vi "Get Square Periphery.vi"(9 "Radius":dbl=1.0, 10 "Neuron Position":i32[](array[numeric])=[3, 2, 7], 11 "Grid Size":i32[](array[numeric])=[10, 10, 10]) -> (3 "Square Periphery":i32[](array[numeric]))   [LabVIEW 2013]
doc: "This algorithm searches for the periphery of the input neuron given the position (x0,y0,z0) and the radius (r) of the neuron.\n The periphery is a square of edge length 6*r. It returns the ids of all the nodes inside the periphery. It takes into acount the limits of the grid (city).\n It includes the id of the node under study"
panel:
  out "No Elements Inside Periphery":i32
  out "Cycles":i32[](array[numeric])
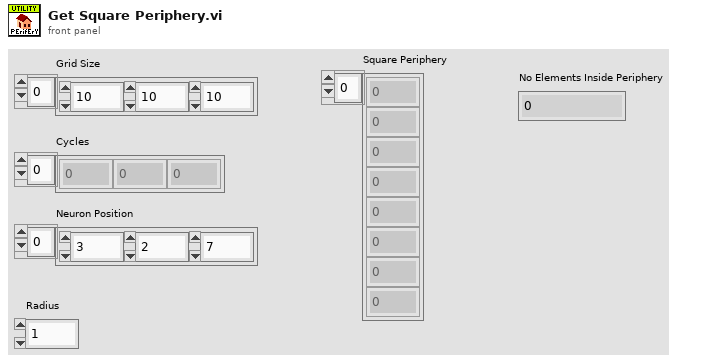
[diagram p1: front panel]
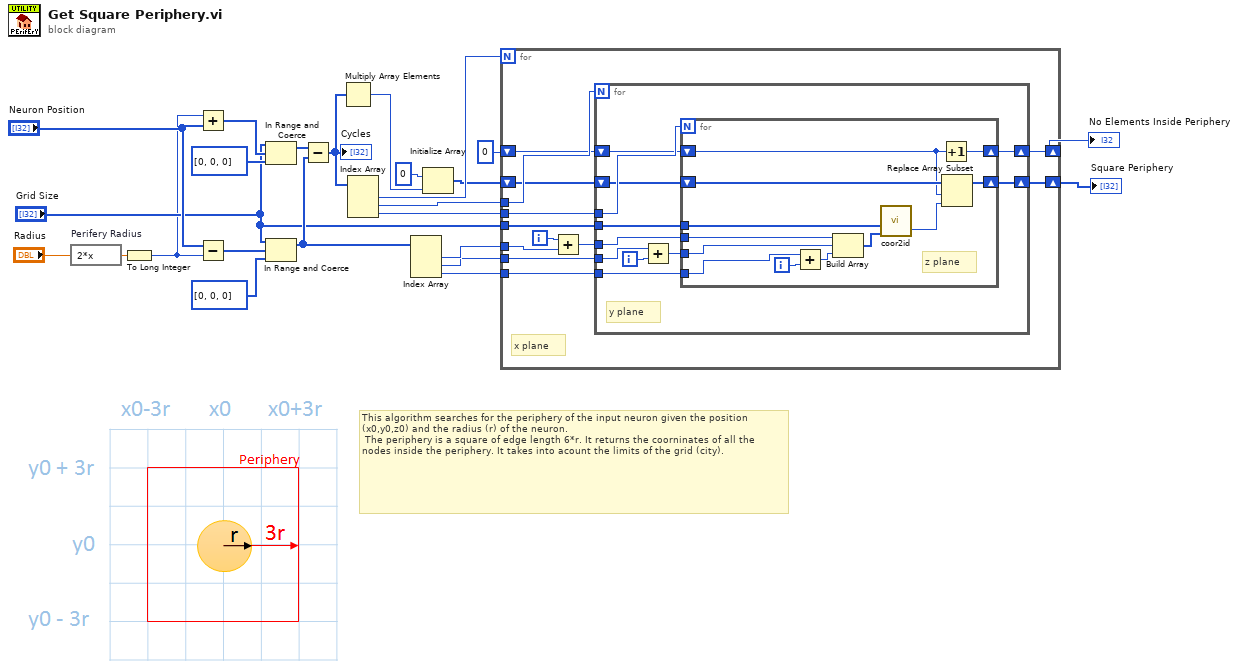
[diagram p0: block diagram]
diagram:
  # "This algorithm searches for the periphery of the input neuron given the position (x0,y0,z0) and the radius (r) of the neuron.\n The periphery is a square of edge length 6*r. It returns the coorninates of all the nodes inside the periphery. It takes into acount the limits of the grid (city)."
  n1 = expression code="2*x" "Perifery Radius"("Radius") -> (w23:dbl)
  n2 = To Long Integer(number=w23) -> (32bit integer=w1:i32)
  n3 = Add(x=w1, y="Neuron Position") -> (x+y=w21:i32[])
  n4 = Subtract(x="Neuron Position", y=w1) -> (x-y=w22:i32[])
  n5 = In Range and Coerce(upper limit="Grid Size", x=w21, lower limit=i32[] [0, 0, 0]) -> (coerced(x)=w19:i32[])  [unwired: 1 out]
  n6 = In Range and Coerce(upper limit="Grid Size", x=w22, lower limit=i32[] [0, 0, 0]) -> (coerced(x)=w16:i32[])  [unwired: 1 out]
  n7 = Subtract(x=w19, y=w16) -> (x-y=w10:i32[])
  "Cycles" <- w10
  n8 = Multiply Array Elements(1:w10) -> (0:w9:i32)
  n9 = Index Array(array=w10) -> (element #1=w18:i32, element #2=w13:i32, element #3=w12:i32)  [unwired: 3 in]
  n10 = Index Array(array=w16) -> (element #1=w15:i32, element #2=w14:i32, element #3=w11:i32)  [unwired: 3 in]
  n11 = Initialize Array(0 ("element"), w9) -> (w6:i32[])
  n12 = for {
    N: w18 -> [_]
    tunnel: w15 -> [w35]
    tunnel: w14 -> [w33]
    tunnel: w13 -> [w32]
    tunnel: w12 -> [w31]
    tunnel: w11 -> [w30]
    shift-right: [w27] -> w5
    shift-left: 0 ("element") -> [w28]
    shift-right: [w26] -> w2
    shift-left: w6 -> [w29]
    tunnel: "Grid Size" -> [w25]
    i -> [w36]
    # "x plane"
    n13 = Add(x=w36, y=w35) -> (x+y=w34:i32)
    n14 = for {
      N: w32 -> [_]
      tunnel: w34 -> [w42]
      tunnel: w33 -> [w46]
      tunnel: w31 -> [w45]
      tunnel: w30 -> [w44]
      shift-right: [w40] -> w27
      shift-left: w28 -> [w41]
      shift-right: [w39] -> w26
      shift-left: w29 -> [w38]
      tunnel: w25 -> [w37]
      i -> [w47]
      # "y plane"
      n15 = Add(x=w46, y=w47) -> (x+y=w43:i32)
      n16 = for {
        N: w45 -> [_]
        tunnel: w44 -> [w59]
        tunnel: w43 -> [w56]
        tunnel: w42 -> [w55]
        shift-right: [w54] -> w40
        shift-left: w41 -> [w51]
        shift-right: [w50] -> w39
        shift-left: w38 -> [w53]
        tunnel: w37 -> [w48]
        i -> [w58]
        # "z plane"
        n17 = Add(x=w59, y=w58) -> (x+y=w57:i32)
        n18 = Build Array(w55, w56, w57) -> (w52:i32[])
        n19 = call "coor2id.vi"("Square Periphery"=w52, "Size(um)"=w48) -> ("Id"=w49:i32)  [unwired: 5 in]
        n20 = Increment(x=w51) -> (x+1=w54:i32)
        n21 = Replace Array Subset(array=w53, new element=w49, index=w51) -> (w50:i32[])
      }
    }
  }
  "No Elements Inside Periphery" <- w5
  "Square Periphery" <- w2
